vi "Make Call.vi"(8 "error in (no error)":errorcluster, 11 "Customer With Phone In":refnum<class "Customer With Phone.lvclass">) -> (0 "error out":errorcluster, 3 "Customer With Phone Out":refnum<class "Customer With Phone.lvclass">)   [LabVIEW 2020, in "Customer With Phone.lvclass"]
uses:
  Customer With Phone.lvclass
  C:/Program Files (x86)/National Instruments/LabVIEW 2020/vi.lib/Astemes/Triarc Framework/Process/Process.lvclass
  <vilib>/Astemes/Triarc Framework/Process/Process.lvclass/Process.ctl
  <vilib>/Astemes/Triarc Framework/Process/Private/SubVIs/Handle Debug Data.vi
  <vilib>/Astemes/Triarc Framework/Logging/Log Debug.vi
  <vilib>/AdvancedString/1D String Array to Delimited String.vi
  <vilib>/Utility/High Resolution Relative Seconds.vi
  <vilib>/Astemes/Triarc Framework/Process/Public/Read Name.vi
  <vilib>/Astemes/Triarc Framework/Callback/Callback.lvclass
  <vilib>/Astemes/Triarc Framework/Process/Process.lvclass
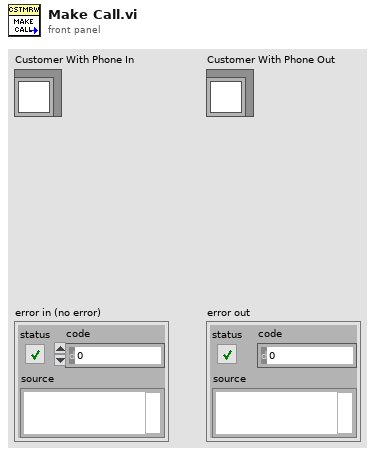
[diagram p1: front panel]
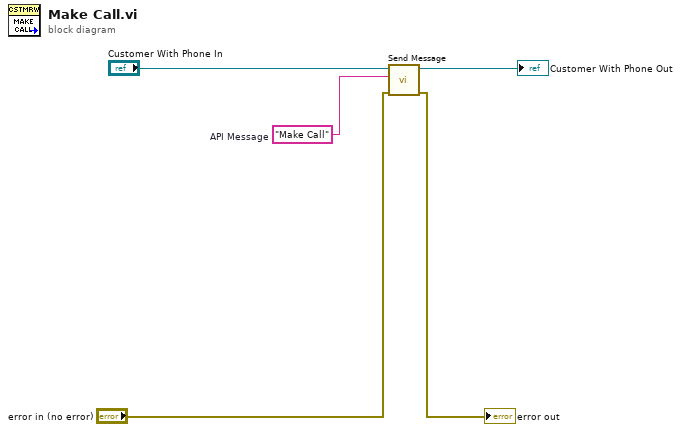
[diagram p0: block diagram]
diagram:
  w2 = "Make Call"  # API Message
  n1 = call <vilib>:"Send Message.vi"("error in (no error)"="error in (no error)", "Message"=w2, "Process In"="Customer With Phone In") -> ("error out"=→"error out":errorcluster, "Process Out"=→"Customer With Phone Out":refnum<class "Customer With Phone.lvclass">)  [unwired: 7 in]
